vi "URAPI_WriteAnalogOut_num.vi"(0 "Variable In":dbl, 3 "URAPI Script":T1={"Script"="", "Whiles"=[], "Ifs"=[], "Supress Err"=TRUE, "Errors"=""}, 4 "Channel":u8) -> (2 "Variable Out":string, 5 "URAPI Script":T1={"Script"="", "Whiles"=[], "Ifs"=[], "Supress Err"=TRUE, "Errors"=""})   [LabVIEW 2012]
doc: "Writes the specified \"Variable in\" value to the specified analog \"Channel\"."
uses:
  <userlib>/BotSpeak/VIs/Direct/URAPI_Control.ctl
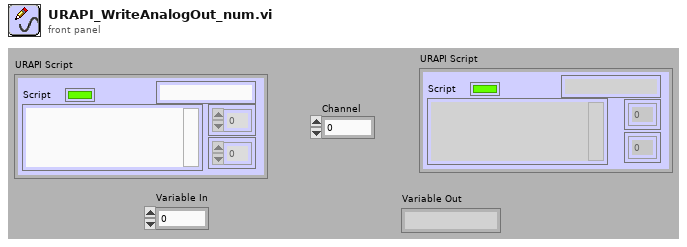
[diagram p1: front panel]
types:
  T1 = typedef "URAPI_Control.ctl" = cluster{"Script":string, "Whiles":u8[], "Ifs":u8[], "Supress Err":bool, "Errors":string}
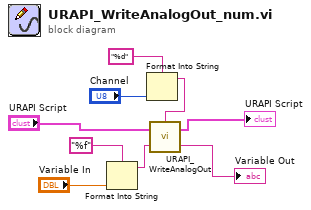
[diagram p0: block diagram]
diagram:
  n1 = Format Into String(format string="%f", "Variable In") -> (resulting string=w1:string)  [unwired: 2 in, 1 out]
  n2 = Format Into String(format string="%d" ("string"), "Channel") -> (resulting string=w4:string)  [unwired: 2 in, 1 out]
  n3 = call <userlib>:"URAPI_WriteAnalogOut.vi"("Variable In"=w1, "URAPI Script"="URAPI Script", "Channel"=w4) -> ("Variable Out"=→"Variable Out":string, "URAPI Script"=→"URAPI Script":T1)  [unwired: 1 in]
